vi "network stream write bulk.vi"(8 "error in (no error)":errorcluster, 10 "Data":fxp<+/-,17,5>[](array[numeric]) format="%#_17g", 11 "endpoint in":refnum<k21>) -> (0 "error out":errorcluster, 3 "endpoint out":refnum<k21>)   [LabVIEW 2024]
uses:
  <resource>/objmgr/ni.dex.rc
panel:
  out "Data sent num":i32
  out "Remaining data num":i32
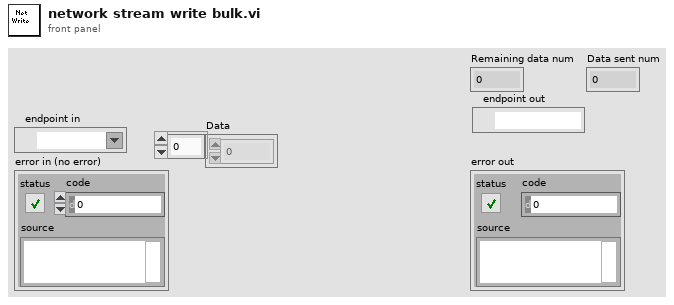
[diagram p1: front panel]
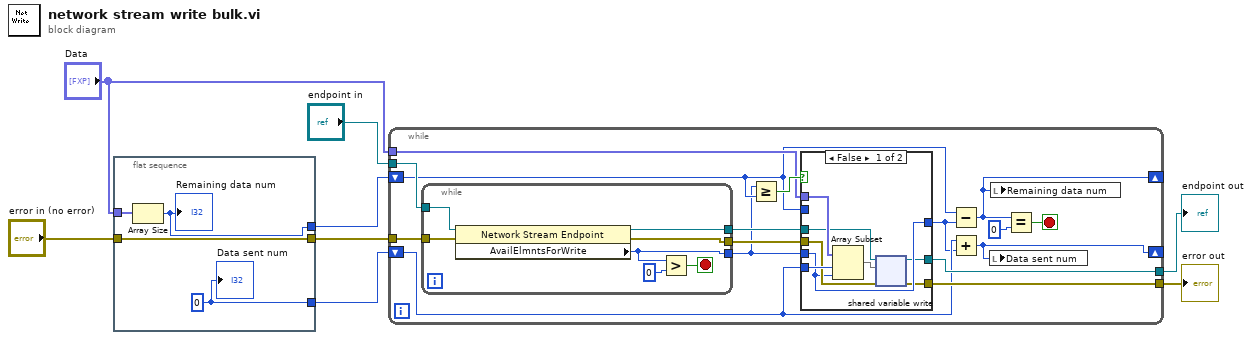
[diagram p0: block diagram]
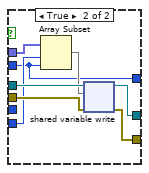
[diagram p2: hidden frame]
diagram:
  n1 = flat-sequence {
    tunnel: "error in (no error)" -> [w12]
    tunnel: [w12] -> w5
    tunnel: "Data" -> [w11]
    tunnel: [w10] -> w3
    tunnel: [w9] -> w1
    frame #0 {
      w9 = 0 ("Data sent")
      n2 = Array Size(array=w11) -> (size(s)=w10:i32)
      "Remaining data num" <- w10
      "Data sent num" <- w9
    }
  }
  n3 = while {
    tunnel: w5 -> [w27]
    tunnel: [w22] -> w7
    tunnel: "endpoint in" -> [w28]
    tunnel: [w21] -> w4
    shift-right: [w17] -> _
    shift-left: w3 -> [w18]
    tunnel: "Data" -> [w23]
    shift-right: [w14] -> _
    shift-left: w1 -> [w16]
    stop <- w19 stop-if-true
    n4 = while {
      tunnel: w28 -> [w51]
      tunnel: w27 -> [w50]
      tunnel: [w47] -> w25
      tunnel: [w46] -> w24
      tunnel: [w45] -> w13
      stop <- w48 stop-if-true
      n5 = property class="Network Stream Endpoint"(reference=w51, error in=w50) -> (reference out=w47:refnum<k21>, error out=w46:errorcluster, "AvailElmntsForWrite"=w45:i32)
      n6 = Greater?(x=w45, y=0) -> (0:w48:bool)
    }
    n7 = Greater Or Equal?(x=w13, y=w18) -> (x >= y?=w26:bool)
    n8 = case shown="False" w26 {
      tunnel: w25 -> [w33 w44]
      tunnel: w24 -> [w32 w43]
      tunnel: w23 -> [w36 w42]
      tunnel: w16 -> [w35 w41]
      tunnel: w18 -> [_ w37]
      tunnel: [w29 w39] -> w22
      tunnel: [w30 w38] -> w21
      tunnel: [w31 w37] -> w15
      tunnel: w13 -> [w31 _]
      frame False {
        n9 = Array Subset(array=w36, index=w35, length=w31) -> (w34:fxp<+/-,17,5>[])
        n10 = shared-variable-write(w33, w32, w34) -> (w30:refnum<k21>, w29:errorcluster)  [unwired: 1 in, 1 out]
      }
      frame True {
        n11 = Array Subset(array=w42, index=w41, length=w37) -> (w40:fxp<+/-,17,5>[])
        n12 = shared-variable-write(w44, w43, w40) -> (w38:refnum<k21>, w39:errorcluster)  [unwired: 1 in, 1 out]
      }
    }
    n13 = Subtract(x=w18, y=w15) -> (x-y=w17:i32)
    n14 = Add(x=w16, y=w15) -> (x+y=w14:i32)
    n15 = local write "Data sent num"(w14) -> ()
    n16 = local write "Remaining data num"(w17) -> ()
    n17 = Equal?(x=w17, y=0) -> (x = y?=w19:bool)
  }
  "error out" <- w7
  "endpoint out" <- w4
